vi "24-bit number to SGL.vi"(9 "Input Valid":bool=TRUE, 10 "Input":fxp<+/-,24,3>) -> (1 "Output Valid":bool=TRUE, 2 "SGL Output":fxp<+,32,32>)   [LabVIEW 2011]
uses:
  <vilib>/rvi/IPIntegrationNode/IPINode_Utilities/niFpgaIPINodeSimCore.vi
  <vilib>/rvi/FXPMathLib/basic elements/FxpDiscreteDelay/XNode/nifxpmath_DiscreteDelay.xnode
  <vilib>/rvi/XilinxIP/XIPIN_XNode/niFpgaXIPIN.xnode
  <userlib>/FPGA Library/Code Development/SGL/Conversions/24-bit to SGL/twofourbittosgl_3410E022421911E643C4BE9C91E41A20.dll
  <vilib>/rvi/IPIntegrationNode/IPINode_Xnode/niFpgaIPINode.xnode
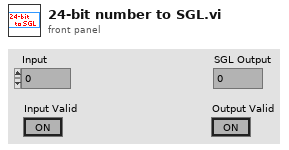
[diagram p1: front panel]
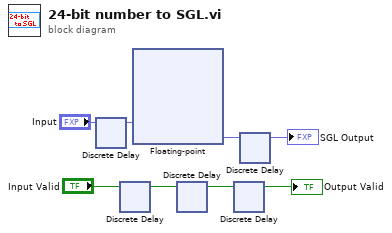
[diagram p0: block diagram]
diagram:
  n1 = xnode "Discrete Delay"("D"="Input") -> ("Q"=w2:fxp<+/-,24,3>)
  n2 = xnode "Discrete Delay"("D"="Input Valid") -> ("Q"=w1:bool)
  n3 = xnode ("Floating-point")("a"=w2) -> ("result"=w7:fxp<+,32,32>)
  n4 = xnode "Discrete Delay"("D"=w1) -> ("Q"=w5:bool)
  n5 = xnode "Discrete Delay"("D"=w5) -> ("Q"=→"Output Valid":bool)
  n6 = xnode "Discrete Delay"("D"=w7) -> ("Q"=→"SGL Output":fxp<+,32,32>)
